vi "timekeeper offset from timeref (g).vi"() -> ()   [LabVIEW 2011, in "EPS_Timekeeper.lvlib"]
uses:
  <vilib>/addons/Electrical Power/Example Support/PMU/Time Keeper/EPS_Timekeeper.lvlib
panel:
  in  "Offset from Timeref (g)":fxp<+/-,21,21>
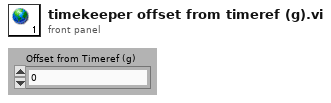
[diagram p1: front panel]
diagram:
